vi "Test Device API.vi"(8 "error in (no error)":errorcluster) -> (0 "error out":errorcluster)   [LabVIEW 2015]
uses:
  Device/Device.lvclass
  <vilib>/addons/_JKI Toolkits/Caraya/classes/Test/Test.lvclass
  <vilib>/addons/_JKI Toolkits/Caraya/classes/Assert/Assert.lvclass
  Window/Window.lvclass
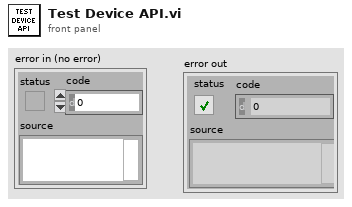
[diagram p1: front panel]
types:
  T1 = typedef "imagedata.ctl" = cluster{"image type":i32, "image depth":i32, "image":u8[], "mask":u8[], "colors":u32[], "Rectangle":cluster{"left":i16, "top":i16, "right":i16, "bottom":i16}}
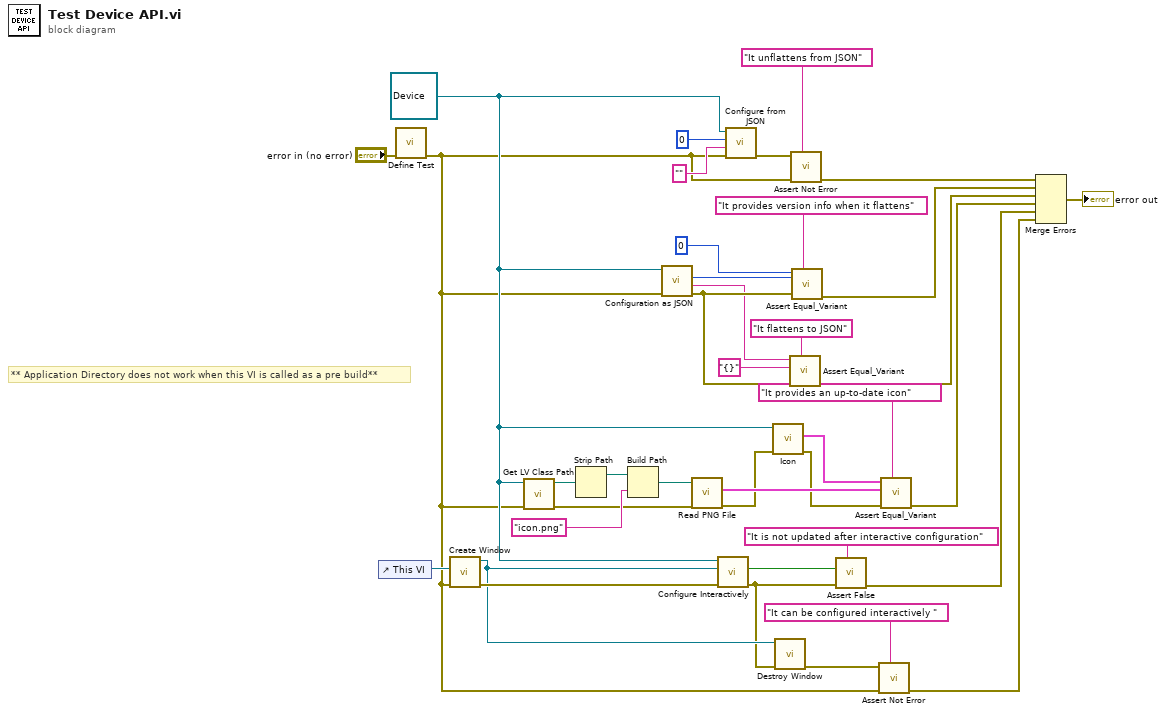
[diagram p0: block diagram]
diagram:
  w9 = refnum<class "Device.lvclass"> refnum ("Device in")
  # "** Application Directory does not work when this VI is called as a pre build**"
  n1 = control-ref of="This VI"() -> (w19:refnum<vi>)
  n2 = call <vilib>:"Define Test.vi"("error in (no error)"="error in (no error)") -> ("error out"=w8:errorcluster)  [unwired: 10 in]
  n3 = call "Create Window.vi"("error in (no error)"=w8, "Window"=w19) -> ("error out"=w18:errorcluster, "Window out"=w17:refnum<class "Window.lvclass">)  [unwired: 8 in]
  n4 = call <vilib>:"Get LV Class Path.vi"("error in (no error)"=w8, "object"=w9) -> ("error out"=w3:errorcluster, "class path"=w6:path)  [unwired: 8 in]
  n5 = Strip Path(path=w6) -> (stripped path=w5:path)  [unwired: 1 out]
  n6 = Build Path(base path=w5, name or relative path="icon.png" ("pattern")) -> (appended path=w2:path)
  n7 = call-dynamic "Configuration as JSON.vi"("error in (no error)"=w8, "Device in"=w9) -> ("error out"=w35:errorcluster, "JSON Data"=w33:string, "Version"=w37:u32)  [unwired: 6 in, 1 out]
  n8 = call <vilib>:"Read PNG File.vi"("error in (no error)"=w3, "path to PNG file"=w2) -> ("error out"=w1:errorcluster, "image data"=w23:T1)  [unwired: 7 in, 1 out]
  n9 = call-dynamic "Configure Interactively.vi"("error in (no error)"=w18, "Parent Window"=w17, "Device in"=w9) -> ("error out"=w12:errorcluster, "Updated"=w14:bool)  [unwired: 6 in, 1 out]
  n10 = call-dynamic "Configure from JSON.vi"("error in (no error)"=w8, "JSON Data"="", "Version"=u32 0, "Device in"=w9) -> ("error out"=w32:errorcluster)  [unwired: 6 in, 1 out]
  n11 = call-dynamic "Icon.vi"("error in (no error)"=w1, "Device in"=w9) -> ("error out"=w22:errorcluster, "Icon"=w7:T1)  [unwired: 7 in, 1 out]
  n12 = call "Destroy Window.vi"("error in (no error)"=w12, "Window in"=w17) -> ("error out"=w16:errorcluster)  [unwired: 9 in]
  n13 = call <vilib>:"Assert Equal_Variant.vi"("Label"="It flattens to JSON", "error in (no error)"=w35, "Y"="{}", "X"=w33) -> ("error out"=w25:errorcluster)  [unwired: 7 in]
  n14 = call <vilib>:"Assert Not Error.vi"("Label"="It unflattens from JSON", "error in (no error)"=w8, "Not Error?"=w32) -> ("error out"=w27:errorcluster)  [unwired: 8 in]
  n15 = call <vilib>:"Assert Equal_Variant.vi"("Label"="It provides version info when it flattens", "error in (no error)"=w35, "Y"=w37, "X"=u32 0) -> ("error out"=w26:errorcluster)  [unwired: 7 in]
  n16 = call <vilib>:"Assert False.vi"("Label"="It is not updated after interactive configuration", "error in (no error)"=w12, "False?"=w14) -> ("error out"=w11:errorcluster)  [unwired: 8 in]
  n17 = call <vilib>:"Assert Not Error.vi"("Label"="It can be configured interactively ", "error in (no error)"=w8, "Not Error?"=w16) -> ("error out"=w10:errorcluster)  [unwired: 8 in]
  n18 = call <vilib>:"Assert Equal_Variant.vi"("Label"="It provides an up-to-date icon", "error in (no error)"=w22, "Y"=w23, "X"=w7) -> ("error out"=w21:errorcluster)  [unwired: 7 in]
  n19 = Merge Errors(w27, w26, w25, w21, w11, w10) -> (→"error out":errorcluster)
